vi "Yes No PopUp Box.vi"(8 "Error In":errorcluster, 9 "Cancel Button Text":string, 10 "Done Button text":string, 11 "Input Message":string="COMMUNICATION METHOD") -> (0 "Error Out":errorcluster, 3 "User DOne":bool)   [LabVIEW 2014]
uses:
  Buttons/Standard button.ctl
  Application Support/Front Panel/Window In Front/Bring Caller to Front.vi
  Application Support/Stop Button/SubVI/Get Stop Button Status.vi
panel:
  in  "Cancel":T1
  out "String":string="COMMUNICATION METHOD"
  in  "Done":T1
  in  "Join Mission":bool
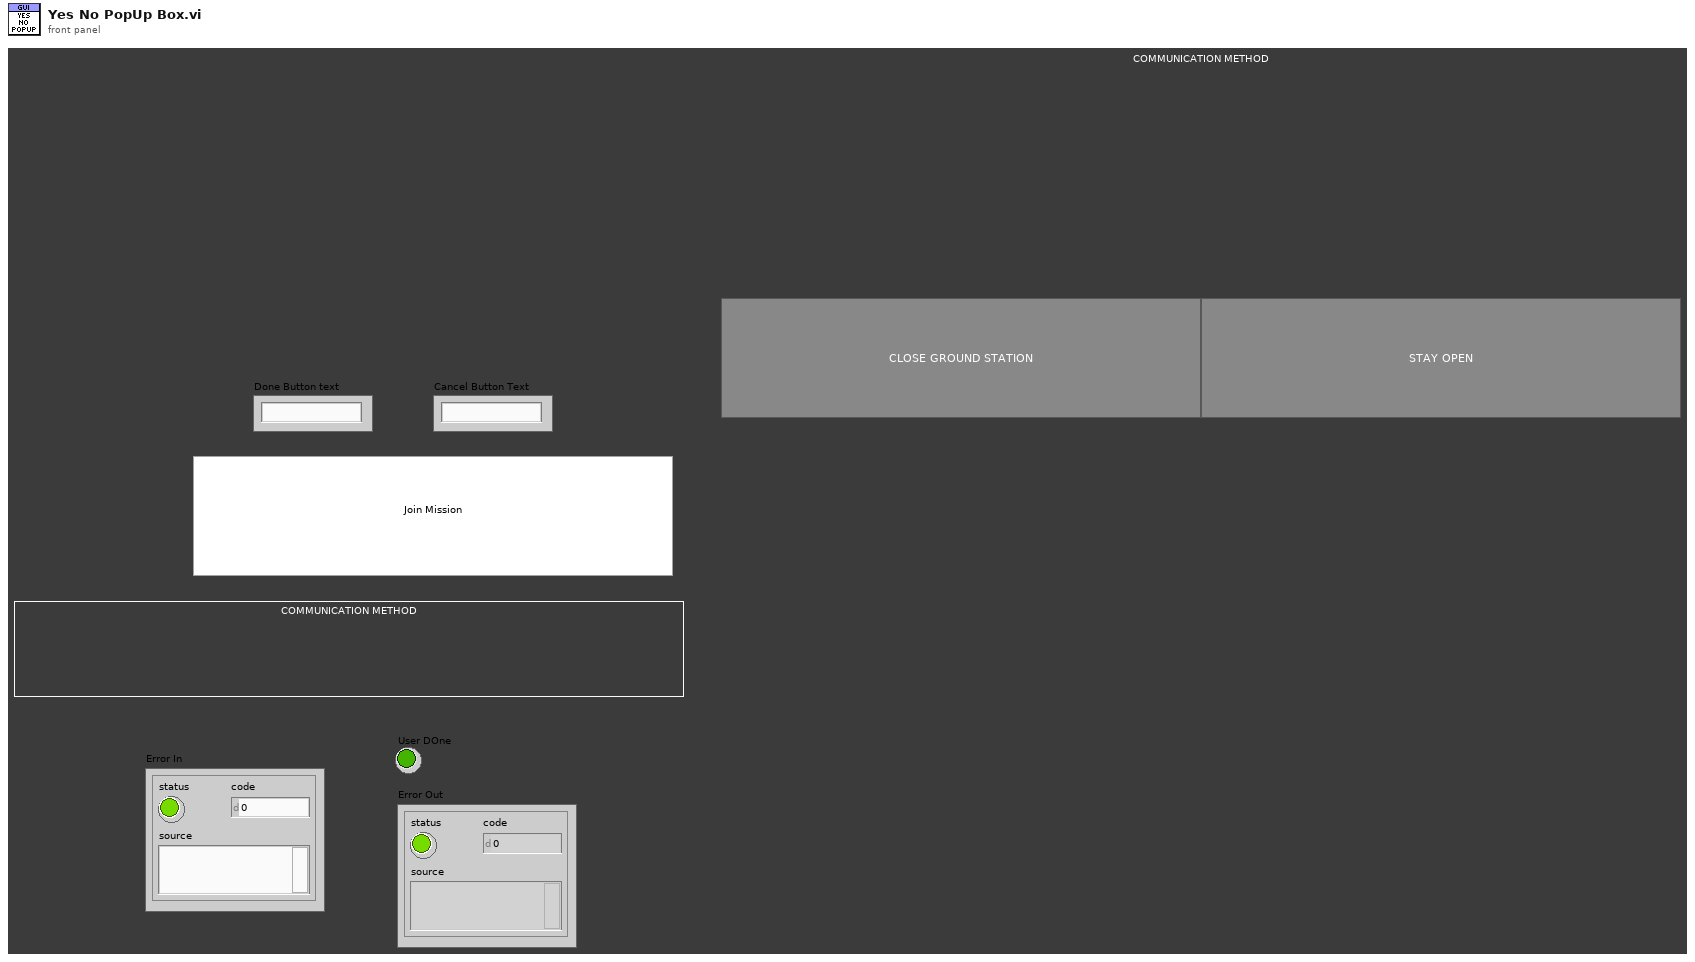
[diagram p1: front panel]
types:
  T1 = typedef "Standard button.ctl" = bool
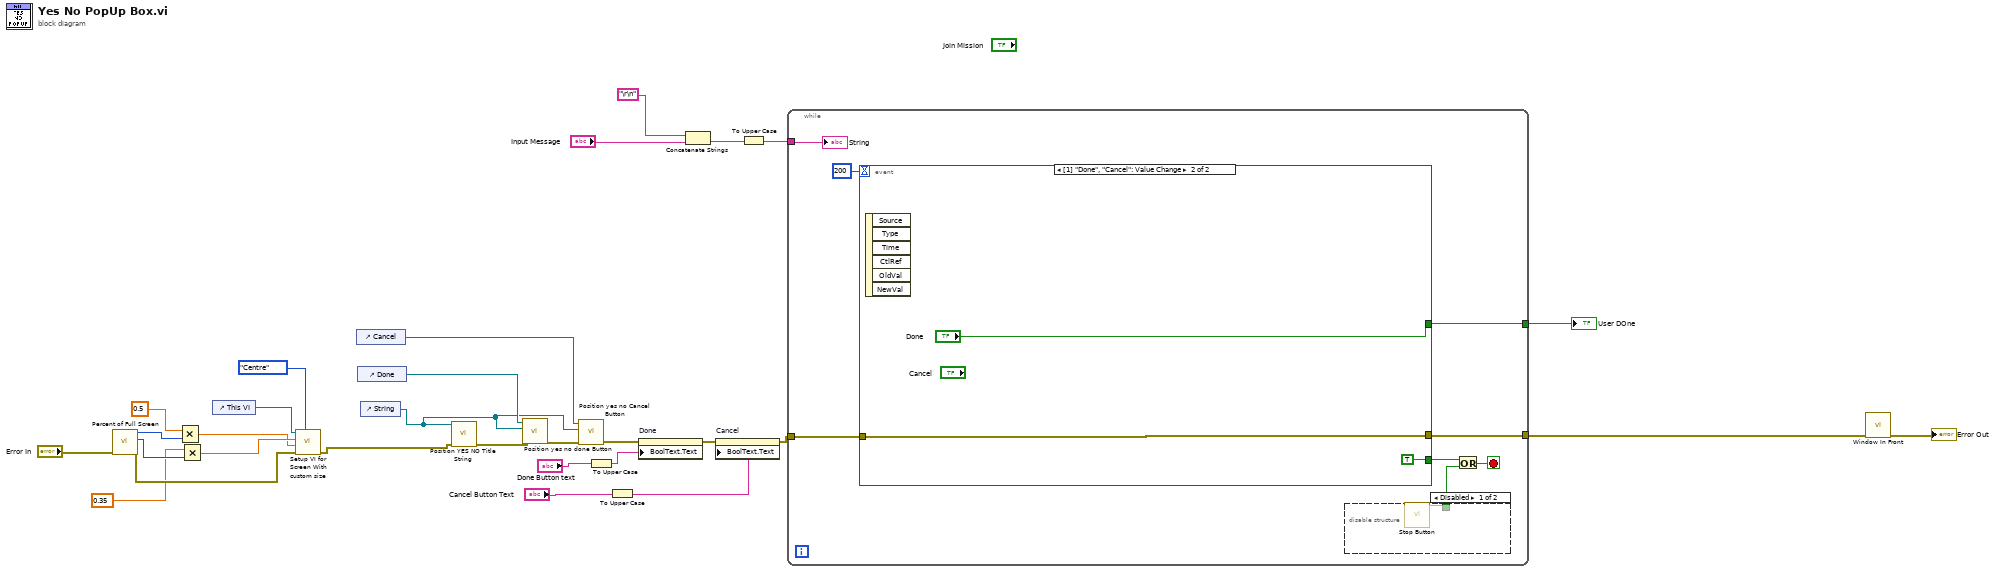
[diagram p0: block diagram]
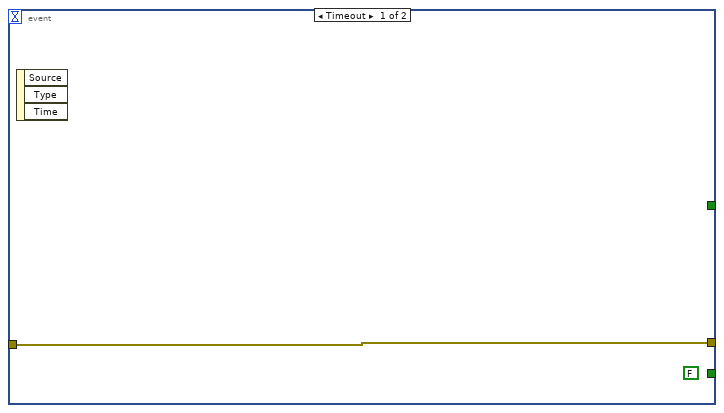
[diagram p3: hidden frame]
diagram:
  n1 = call "Percent of Full Screen.vi"("error in (no error)"="Error In") -> ("error out"=w20:errorcluster, "Bottom"=w24:i16, "Right"=w25:i16)  [unwired: 8 in]
  n2 = Multiply(x=0.5, y=w25) -> (x*y=w21:dbl)
  n3 = Multiply(x=0.35, y=w24) -> (x*y=w22:dbl)
  n4 = control-ref of="This VI"() -> (w27:refnum<vi>)
  n5 = call "Setup VI for Screen With custom size.vi"("Position"=enum16{"Top Left", "Centre"}."Centre", "Error In"=w20, "Width"=w21, "Height"=w22, "This VI"=w27) -> ("Error Out"=w19:errorcluster)  [unwired: 5 in, 1 out]
  n6 = control-ref of="Cancel"() -> (w14:refnum<vi>)
  n7 = control-ref of="Done"() -> (w17:refnum<vi>)
  n8 = control-ref of="String"() -> (w15:refnum<vi>)
  n9 = call "Position YES NO Title String.vi"("error in (no error)"=w19, "String Ref"=w15) -> ("error out"=w18:errorcluster)  [unwired: 9 in]
  n10 = call "Position yes no done Button.vi"("error in (no error)"=w18, "Message"=w15, "Button Ref"=w17) -> ("error out"=w16:errorcluster)  [unwired: 8 in]
  n11 = call "Position yes no Cancel Button.vi"("error in (no error)"=w16, "Message"=w15, "Button Ref"=w14) -> ("error out"=w10:errorcluster)  [unwired: 8 in]
  n12 = To Upper Case(1:"Done Button text") -> (0:w1:string)
  n13 = To Upper Case(1:"Cancel Button Text") -> (0:w3:string)
  n14 = property on="Done" class="Bool"(error in=w10, "BoolText.Text"=w1) -> (error out=w9:errorcluster)  [unwired: 1 in, 1 out]
  n15 = Concatenate Strings("\r\n", "Input Message") -> (w6:string)
  n16 = property on="Cancel" class="Bool"(error in=w9, "BoolText.Text"=w3) -> (error out=w8:errorcluster)  [unwired: 1 in, 1 out]
  n17 = To Upper Case(1:w6) -> (0:w5:string)
  n18 = while {
    tunnel: w8 -> [w35]
    tunnel: [w34] -> w29
    tunnel: w5 -> [w32]
    tunnel: [w31] -> w7
    stop <- w37 stop-if-true
    n19 = event shown="[1] \"Done\", \"Cancel\": Value Change" {
      selector: _ -> [_ _]
      dyn-events: _ -> [_ _]
      timeout: 200 -> [_ _]
      tunnel: [_ TRUE ("x")] -> w36
      tunnel: w35 -> [w40 w43]
      tunnel: [w40 w43] -> w34
      tunnel: [_ "Done"] -> w31
      event Timeout {
        (unwired) FALSE ("x")
        n20 = event-data() -> ()  [unwired: 1 in, 3 out]
      }
      event Value Change {
        n21 = event-data() -> ()  [unwired: 1 in, 6 out]
      }
    }
    n22 = disable-structure shown="Disabled" {
      disable-tunnel: [w39 _] -> w38
      frame Disabled {
        n23 = call-poly "Stop Button.vi"() -> ("Stop ButtonOut"=w39:bool)  [unwired: 10 in, 1 out]
      }
      frame Enabled {
      }
    }
    n24 = Or(x=w36, y=w38) -> (x .or. y?=w37:bool)
    "String" <- w32
  }
  "User DOne" <- w7
  n25 = call-poly "Window In Front.vi"("Error In"=w29) -> ("Error Out"=→"Error Out":errorcluster)  [unwired: 10 in]
